vi "ConfigParseMicroscope.vi"(8 "error in (no error)":errorcluster, 10 "Config Refnum in":refnum<k20>) -> (0 "error out":errorcluster, 3 "Configuration Array":string[][](array[string]))   [LabVIEW 2018, in "Config.lvlib"]
uses:
  Config.lvlib
  <vilib>/xml/NI_XML.lvlib
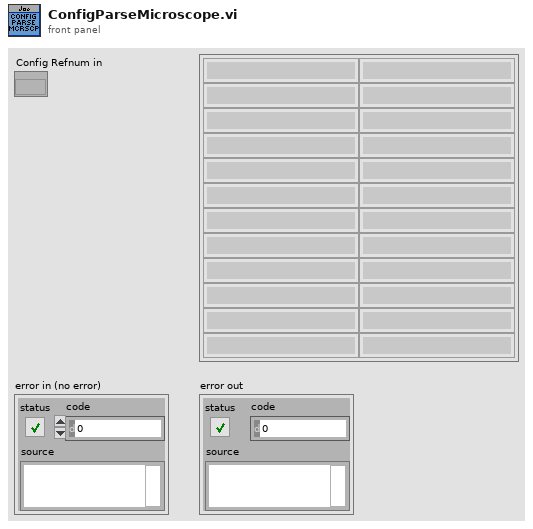
[diagram p1: front panel]
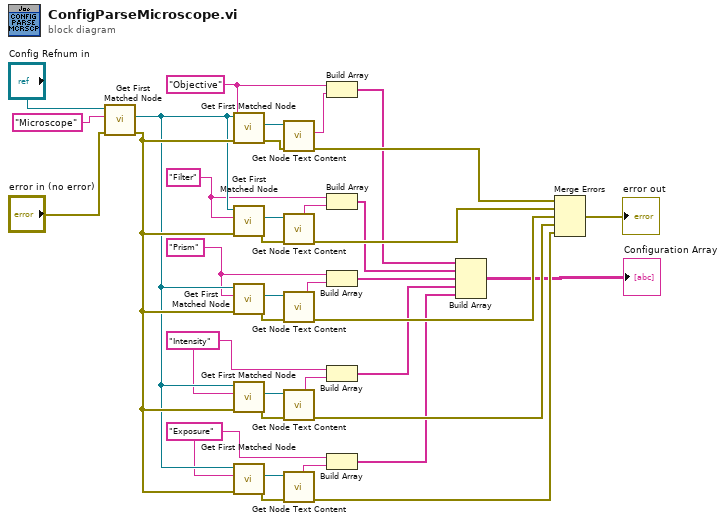
[diagram p0: block diagram]
diagram:
  w18 = "Exposure" ("XPath expression")
  w12 = "Intensity" ("XPath expression")
  w9 = "Prism" ("XPath expression")
  w6 = "Filter" ("XPath expression")
  w2 = "Objective" ("XPath expression")
  n1 = call <vilib>:"Get First Matched Node.vi"("error in (no error)"="error in (no error)", "XPath expression"="Microscope", "node in"="Config Refnum in") -> ("error out"=w37:errorcluster, "node result"=w30:refnum<k20>)  [unwired: 6 in, 1 out]
  n2 = call <vilib>:"Get First Matched Node.vi"("error in (no error)"=w37, "XPath expression"=w2, "node in"=w30) -> ("error out"=w22:errorcluster, "node result"=w1:refnum<k20>)  [unwired: 6 in, 1 out]
  n3 = call <vilib>:"Get First Matched Node.vi"("error in (no error)"=w37, "XPath expression"=w6, "node in"=w30) -> ("error out"=w23:errorcluster, "node result"=w5:refnum<k20>)  [unwired: 6 in, 1 out]
  n4 = call <vilib>:"Get First Matched Node.vi"("error in (no error)"=w37, "XPath expression"=w9, "node in"=w30) -> ("error out"=w24:errorcluster, "node result"=w8:refnum<k20>)  [unwired: 6 in, 1 out]
  n5 = call <vilib>:"Get First Matched Node.vi"("error in (no error)"=w37, "XPath expression"=w12, "node in"=w30) -> ("error out"=w25:errorcluster, "node result"=w11:refnum<k20>)  [unwired: 6 in, 1 out]
  n6 = call <vilib>:"Get First Matched Node.vi"("error in (no error)"=w37, "XPath expression"=w18, "node in"=w30) -> ("error out"=w26:errorcluster, "node result"=w17:refnum<k20>)  [unwired: 6 in, 1 out]
  n7 = call <vilib>:"Get Node Text Content.vi"("error in (no error)"=w22, "node in"=w1) -> ("error out"=w31:errorcluster, "node text"=w3:string)  [unwired: 7 in, 1 out]
  n8 = call <vilib>:"Get Node Text Content.vi"("error in (no error)"=w23, "node in"=w5) -> ("error out"=w32:errorcluster, "node text"=w7:string)  [unwired: 7 in, 1 out]
  n9 = call <vilib>:"Get Node Text Content.vi"("error in (no error)"=w24, "node in"=w8) -> ("error out"=w33:errorcluster, "node text"=w10:string)  [unwired: 7 in, 1 out]
  n10 = call <vilib>:"Get Node Text Content.vi"("error in (no error)"=w25, "node in"=w11) -> ("error out"=w34:errorcluster, "node text"=w13:string)  [unwired: 7 in, 1 out]
  n11 = call <vilib>:"Get Node Text Content.vi"("error in (no error)"=w26, "node in"=w17) -> ("error out"=w35:errorcluster, "node text"=w19:string)  [unwired: 7 in, 1 out]
  n12 = Build Array(w2, w3) -> (w4:string[])
  n13 = Build Array(w6, w7) -> (w14:string[])
  n14 = Build Array(w9, w10) -> (w15:string[])
  n15 = Build Array(w12, w13) -> (w20:string[])
  n16 = Build Array(w18, w19) -> (w21:string[])
  n17 = Build Array(w4, w14, w15, w20, w21) -> (→"Configuration Array":string[][])
  n18 = Merge Errors(w31, w32, w33, w34, w35) -> (→"error out":errorcluster)
